vi "Get Key From INI File.vi"(8 "error in (no error)":errorcluster, 9 "keyName":string, 10 "sectionName":string, 11 "Sections in":refnum<k24>) -> (0 "error out":errorcluster, 2 "keyValue":string, 3 "Sections out":refnum<k24>)   [LabVIEW 2015]
uses:
  C:/C-BOX_DoIP/Utilities/dotNET/C-BOX_DoIP/INIFileParser.dll
  C-BOX_DoIP/Utilities/dotNET/C-BOX_DoIP/INIFileParser.dll
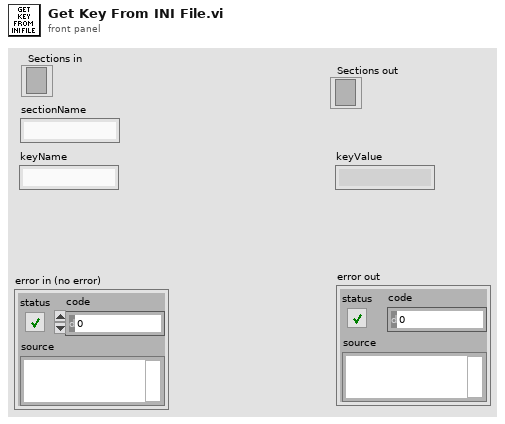
[diagram p1: front panel]
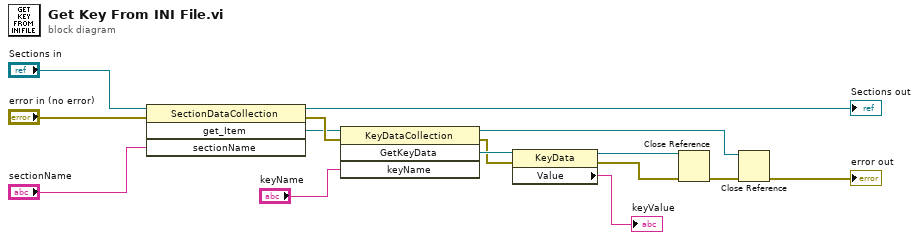
[diagram p0: block diagram]
diagram:
  n1 = invoke class="SectionDataCollection" method="get_Item"(reference="Sections in", error in="error in (no error)", "sectionName"="sectionName") -> (reference out=→"Sections out":refnum<k24>, error out=w14:errorcluster, "get_Item"=w13:refnum<k24>)  [unwired: 1 in, 1 out]
  n2 = invoke class="KeyDataCollection" method="GetKeyData"(reference=w13, error in=w14, "keyName"="keyName") -> (reference out=w3:refnum<k24>, error out=w8:errorcluster, "GetKeyData"=w15:refnum<k24>)  [unwired: 1 in, 1 out]
  n3 = property class="KeyData"(reference=w15, error in=w8) -> (reference out=w6:refnum<k24>, error out=w5:errorcluster, "Value"=→"keyValue":string)
  n4 = Close Reference(reference=w6, error in (no error)=w5) -> (error out=w4:errorcluster)
  n5 = Close Reference(reference=w3, error in (no error)=w4) -> (error out=→"error out":errorcluster)
